vi "Coordinate Array Constants.vi"(10 "Numeric":i32) -> (3 "Axis Positions":dbl[](array[numeric]))   [LabVIEW 2013]
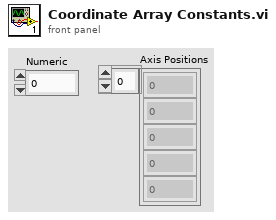
[diagram p1: front panel]
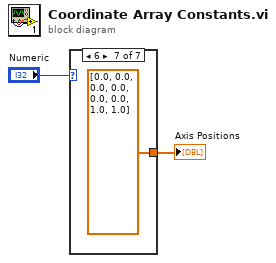
[diagram p0: block diagram]
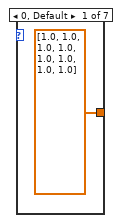
[diagram p2: hidden frame]
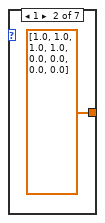
[diagram p3: hidden frame]
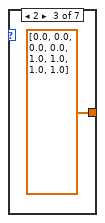
[diagram p4: hidden frame]
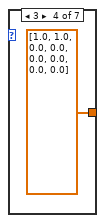
[diagram p5: hidden frame]
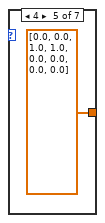
[diagram p6: hidden frame]
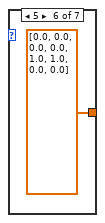
[diagram p7: hidden frame]
diagram:
  n1 = case shown="6" "Numeric" {
    tunnel: [dbl[] [1.0, 1.0, 1.0, 1.0, 1.0, 1.0, 1.0, 1.0] dbl[] [1.0, 1.0, 1.0, 1.0, 0.0, 0.0, 0.0, 0.0] dbl[] [0.0, 0.0, 0.0, 0.0, 1.0, 1.0, 1.0, 1.0] dbl[] [1.0, 1.0, 0.0, 0.0, 0.0, 0.0, 0.0, 0.0] dbl[] [0.0, 0.0, 1.0, 1.0, 0.0, 0.0, 0.0, 0.0] dbl[] [0.0, 0.0, 0.0, 0.0, 1.0, 1.0, 0.0, 0.0] dbl[] [0.0, 0.0, 0.0, 0.0, 0.0, 0.0, 1.0, 1.0]] -> w1
    frame 0, Default {
    }
    frame 1 {
    }
    frame 2 {
    }
    frame 3 {
    }
    frame 4 {
    }
    frame 5 {
    }
    frame 6 {
    }
  }
  "Axis Positions" <- w1
